vi "AutoROI_Setting_UI.vi"(6 "Root":path, 7 "ProjectName":string, 8 "error in (no error)":errorcluster, 11 "Vision_Image":T4(plugin-control)) -> (0 "error out":errorcluster)   [LabVIEW 2019]
uses:
  Controls/AutoROIUI.ctl
  <vilib>/Utility/miscctls.llb/LVPointTypeDef.ctl
  Controls/AutoROIMode.ctl
  <vilib>/vision/Image Controls.llb/IMAQ Image.ctl
  Controls/ROI_List_Action.ctl
  Controls/AutoROIPage.ctl
panel:
  in  "ReadImage":bool
  in  "ROI List":i32[](listbox)
  out "ModeTab":T1
  in  "Numbers":i32=1 min=1 step=1
  in  "ROIDim":T2={"X Pitch"=200, "X Numbers"=1, "Y Pitch"=150, "Y Numbers"=1} {"X Pitch" min=1 step=1; "X Numbers" min=1 step=1; "Y Numbers" min=1 step=1; "Y Pitch" min=1 step=1}
  in  "Step":i32(ring)=1 items=["1 pixel"=1, "10 pixel"=10, "100 pixel"=100]
  in  "X+":bool
  in  "X-":bool
  in  "Y-":bool
  in  "Y+":bool
  in  "Add":bool
  in  "Mode":T3
  in  "Cancel":bool
  in  "OK":bool
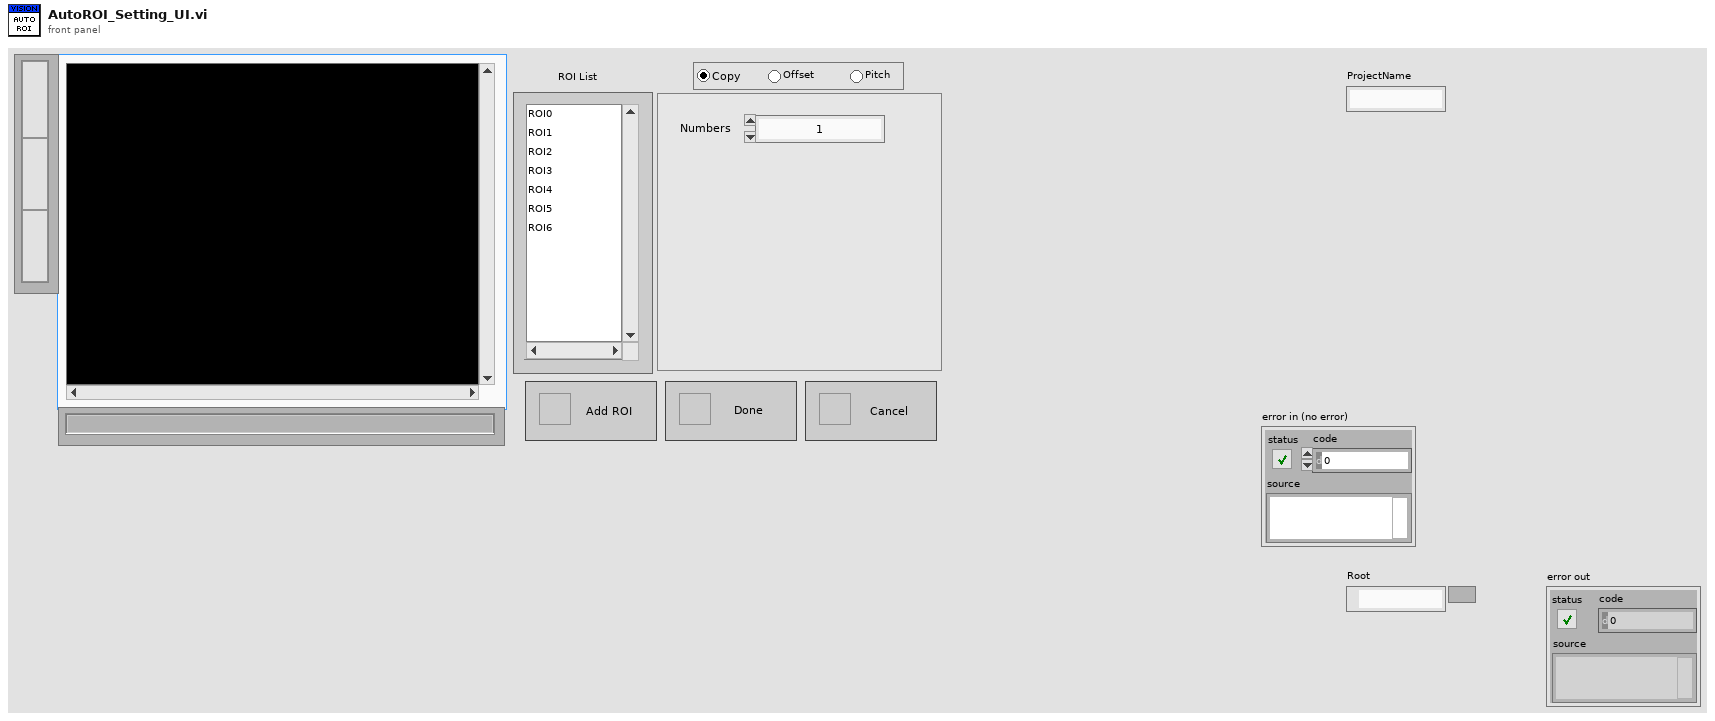
[diagram p1: front panel]
types:
  T1 = typedef "AutoROIPage.ctl" = enum32{"Copy", "Pitch", "Offset"}
  T2 = cluster{"X Pitch":i32, "X Numbers":i32, "Y Pitch":i32, "Y Numbers":i32}
  T3 = typedef "AutoROIMode.ctl" = enum32{"Copy", "Pitch", "Offset"}
  T4 = typedef "IMAQ Image.ctl" = refnum<image>
  T5 = typedef "LVPointTypeDef.ctl" = cluster{"Horizontal":i16, "Vertical":i16}
  T6 = typedef "AutoROIUI.ctl" = cluster{"Message":enum16{"Initialize", "UpdateROIList", "UpdateROI", "Add", "Move", "OK", "Cancel", "Exit"}, "Data":variant}
  T7 = enum8{"Enabled", "Disabled", "Disabled and Grayed Out"}
  T8 = typedef "ROI_List_Action.ctl" = enum16{"Init", "Add ROI", "Delete ROI", "Get All ROI", "Get Specific ROI", "Set Analysis Setting", "Set Process Setting", "Replace All Entries", "ROIEntryBackup", "ROIEntryBackupClear", "ROIEntryReturn"}
  T9 = cluster{"ID":enum32{"External", "Internal"}, "Type":i32, "Coordinates":i32[]}
  T10 = typedef "ROI Descriptor" = cluster{"Global Rectangle":i32[], "Contours":cluster{"ID":enum32{"External", "Internal"}, "Type":u32, "Coordinates":i32[]}[]}
  T11 = enum16{"Initialize", "UpdateROIList", "UpdateROI", "Add", "Move", "OK", "Cancel", "Exit"}
  T12 = typedef "Image Type" = u32
  T13 = typedef "Vision_DataEntry.ctl" = cluster{"vROIName":string, "vROIContour":cluster{"Contour Type":u32, "ROI Type":u32, "Points":i32[]}, "ProcessSetting":T14[], "Analysis_Setting":T16}
  T14 = typedef "Process_Setting.ctl" = cluster{"Enum_PreProcess":T15, "Parameter":string}
  T15 = typedef "VisionProcessName.ctl" = enum16{"*CamParameter*", "CamAttributes", "*Preprocess*", "CG_Brightness", "C_Plane Extraction", "C_Threshold", "G_Lookup Table", "G_Threshold"}
  T16 = typedef "Analysis_Setting.ctl" = cluster{"PreProcess":T17, "Parameter":string}
  T17 = typedef "VisionProcessName.ctl" = enum16{"*CamParameter*", "CamAttributes", "*Preprocess*", "CG_Brightness", "C_Plane Extraction", "C_Threshold", "G_Lookup Table", "G_Threshold", "B_Image Inversion", "*Algorithm*", "CG_Histogram", "C_Color Matching", "C_Color Pattern Matching", "G_PatternMatch", "CG_Find Straight Edge", "CG_Adv. Find Straight Edge", "CG_Find Circular Edge", "G_Max Clamp", "G_Clamp (Rake)", "G_Pattern Matching"}
  T18 = cluster{"Points[0]":i32, "Points[1]":i32, "Points[2]":i32, "Points[3]":i32}
  T19 = cluster{"ID":enum32{"External", "Internal"}, "Type":i32, "Coordinates":i32[]}[]
  T20 = typedef "Vision_DataEntry.ctl" = cluster{"vROIName":string, "vROIContour":cluster{"Contour Type":u32, "ROI Type":u32, "Points":i32[]}, "ProcessSetting":T14[], "Analysis_Setting":T21}
  T21 = typedef "Analysis_Setting.ctl" = cluster{"PreProcess":T22, "Parameter":string}
  T22 = typedef "V_Analysis_Type.ctl" = enum16{"None", "C_Color Pattern Matching", "G_PatternMatching", "G_ShapeDectect", "G_GeometricMatch", "B_Area Check"}
  T23 = cluster{"ID":enum32{"External", "Internal"}, "Type":u32, "Coordinates":i32[]}[]
  T24 = cluster{"ID":enum32{"External", "Internal"}, "Type":u32, "Coordinates":i32[]}
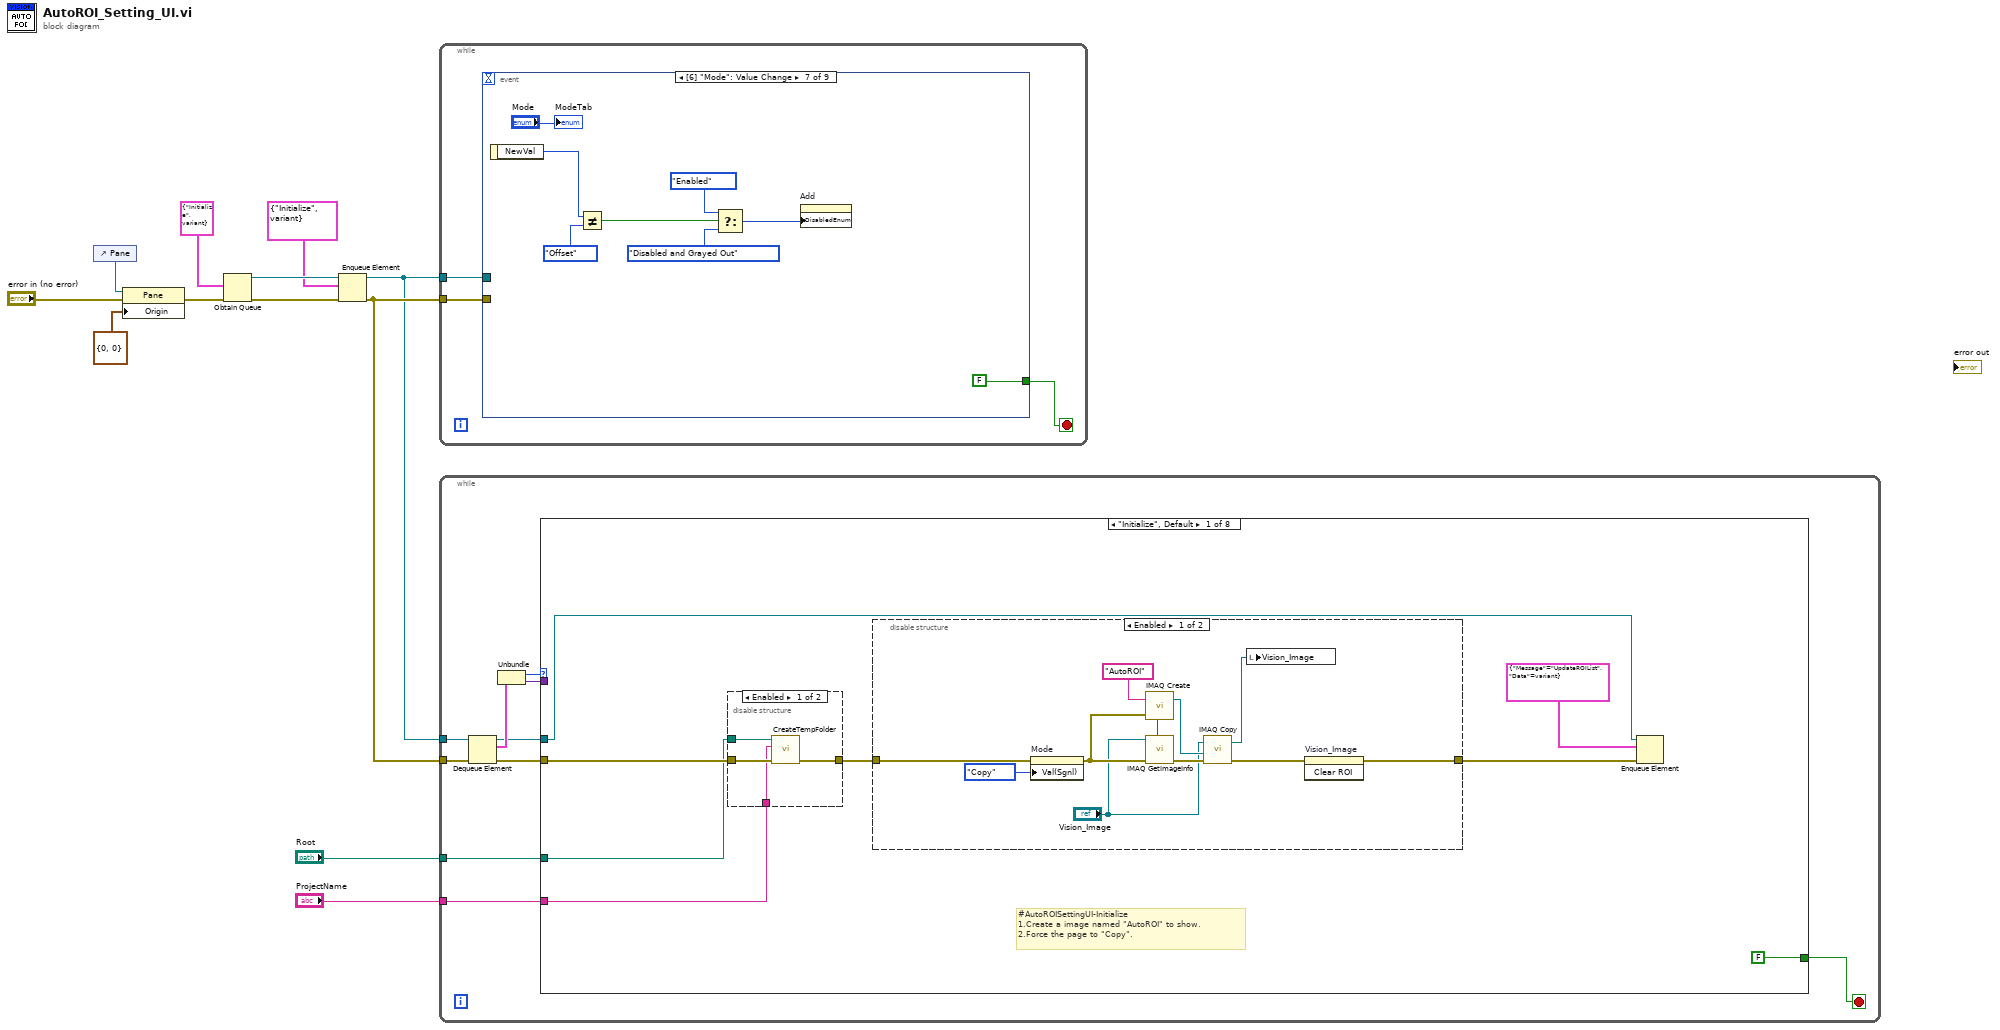
[diagram p0: block diagram]
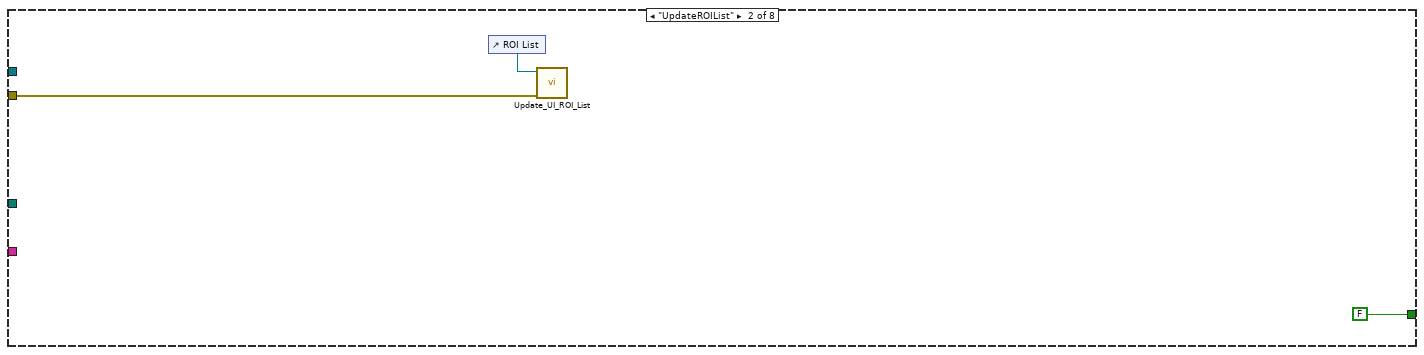
[diagram p4: hidden frame]
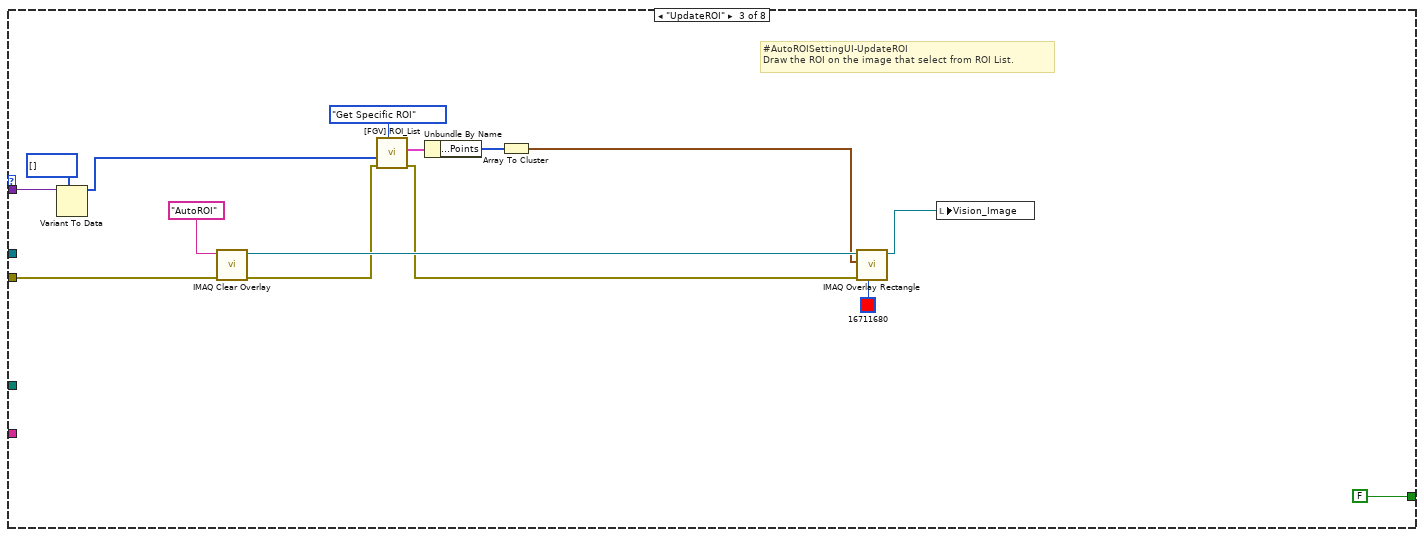
[diagram p5: hidden frame]
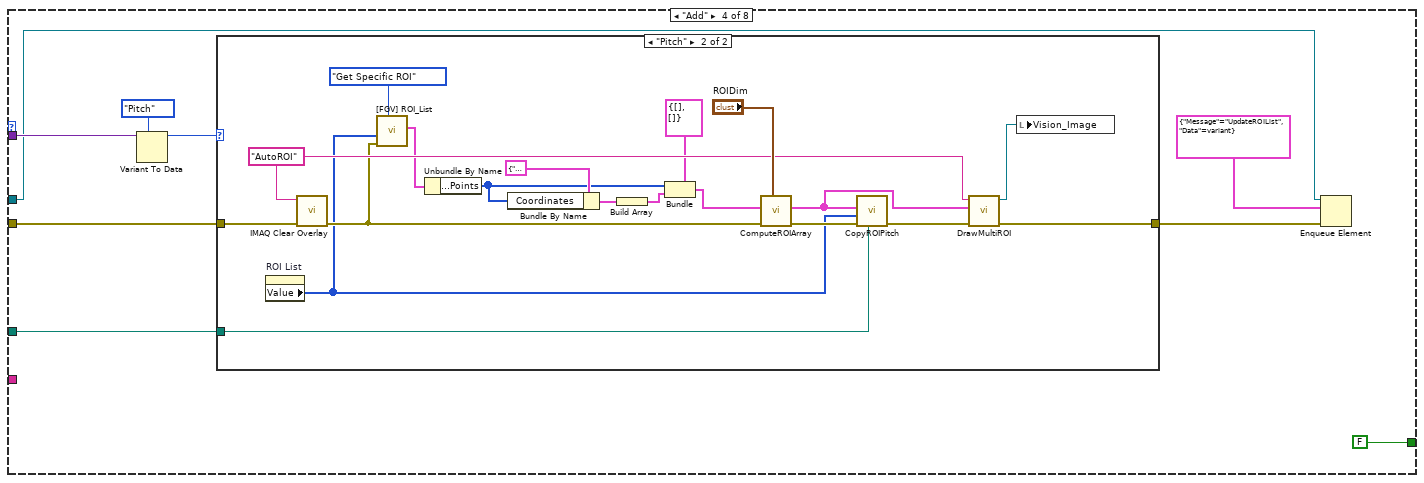
[diagram p6: hidden frame]
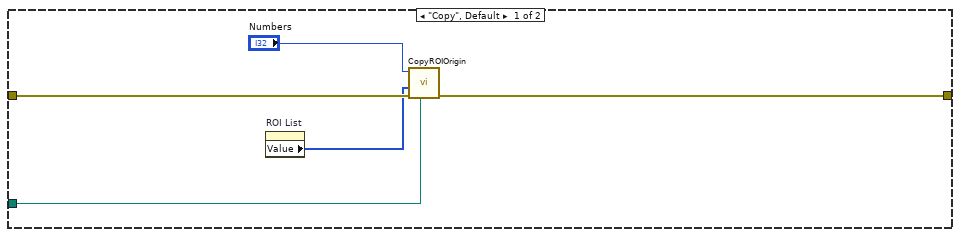
[diagram p7: hidden frame]
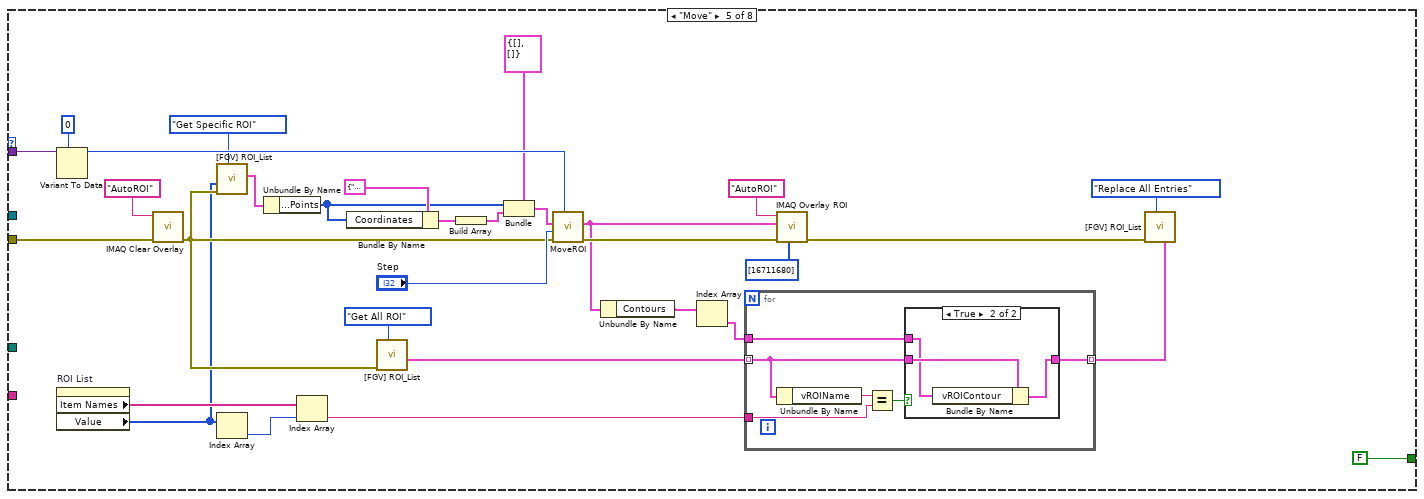
[diagram p8: hidden frame]
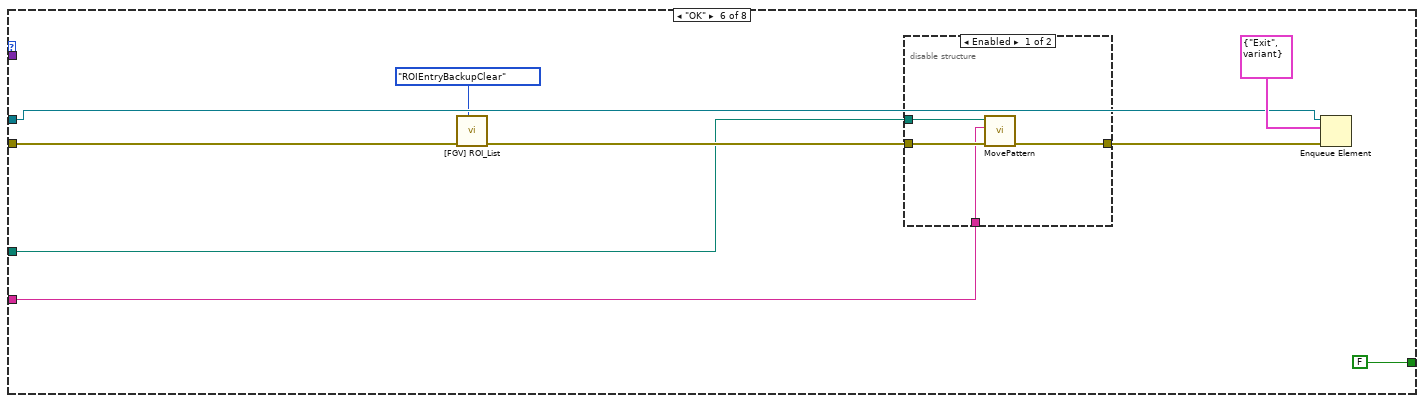
[diagram p10: hidden frame]
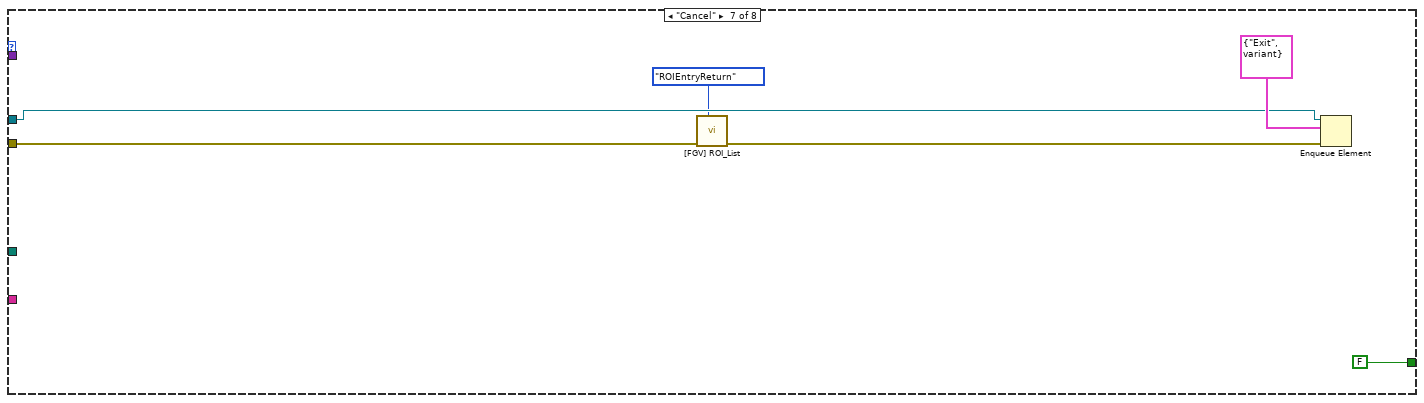
[diagram p12: hidden frame]
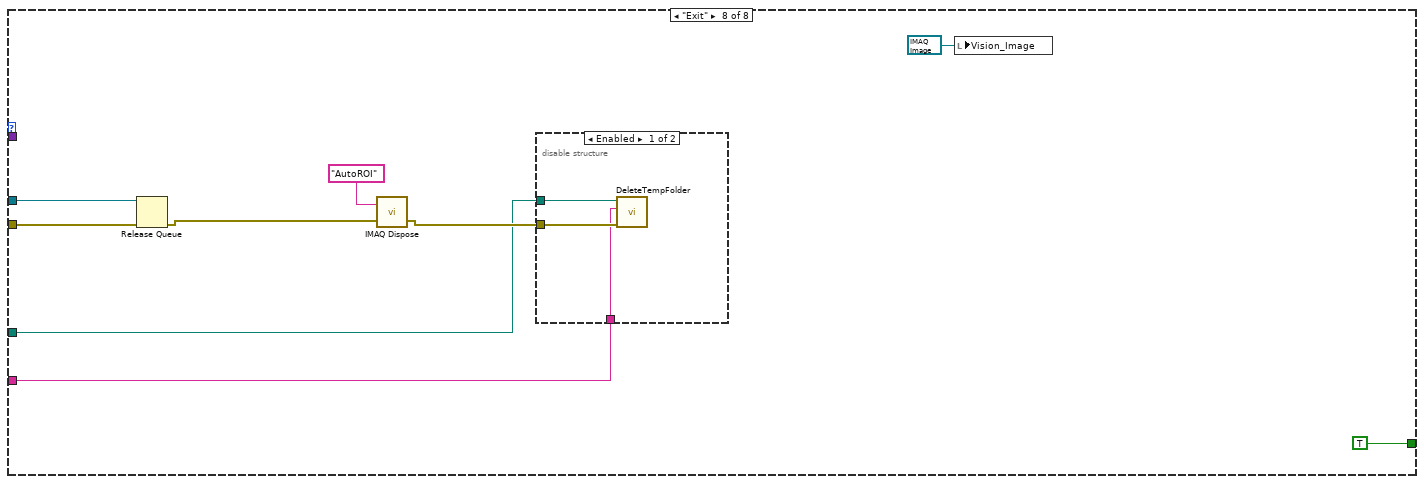
[diagram p13: hidden frame]
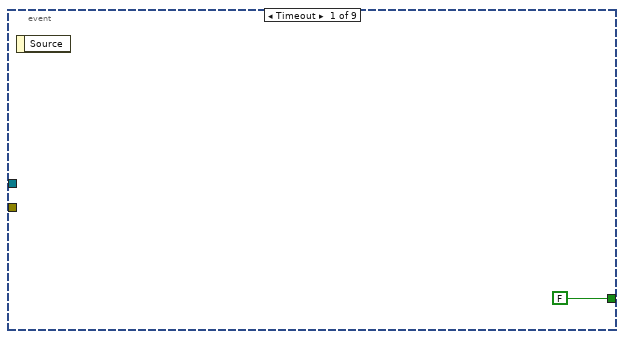
[diagram p15: hidden frame]
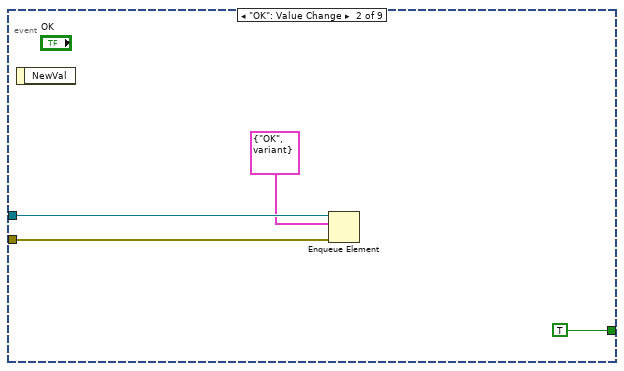
[diagram p16: hidden frame]
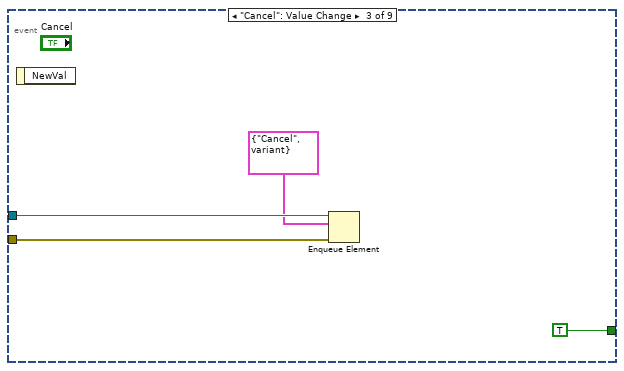
[diagram p17: hidden frame]
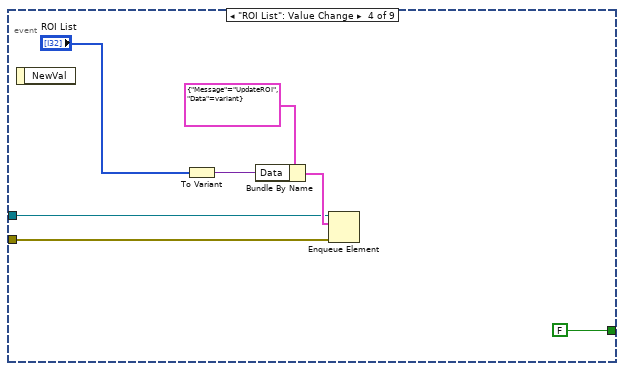
[diagram p18: hidden frame]
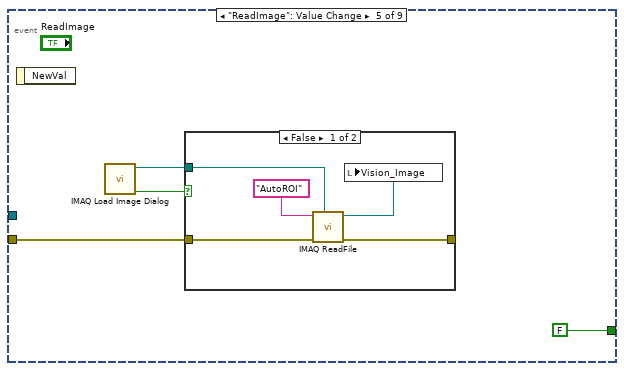
[diagram p19: hidden frame]
diagram:
  n1 = control-ref of="Pane"() -> (w6:refnum<vi>)
  n2 = property class="Pane"(reference=w6, error in="error in (no error)", "Origin"=T5 {"Horizontal"=0, "Vertical"=0}) -> (error out=w5:errorcluster)  [unwired: 1 out]
  n3 = Obtain Queue(element data type=T6 {"Message"=enum."Initialize", "Data"=variant} ("AutoROIUI"), error in (no error)=w5) -> (queue out=w12:refnum<queue>, error out=w11:errorcluster)  [unwired: 3 in, 1 out]
  n4 = Enqueue Element(queue=w12, element=T6 {"Message"=enum."Initialize", "Data"=variant}, error in (no error)=w11) -> (queue out=w7:refnum<queue>, error out=w8:errorcluster)  [unwired: 1 in, 1 out]
  n5 = while {
    tunnel: w7 -> [w14]
    tunnel: w8 -> [w13]
    stop <- w15 stop-if-true
    n6 = event shown="[6] \"Mode\": Value Change" {
      selector: _ -> [_ _ _ _ _ _ _ _ _]
      dyn-events: _ -> [_ _ _ _ _ _ _ _ _]
      timeout: _ -> [_ _ _ _ _ _ _ _ _]
      tunnel: [FALSE TRUE TRUE FALSE FALSE _ FALSE FALSE FALSE] -> w15
      tunnel: w14 -> [_ w19 w23 w27 _ w43 _ w65 w73]
      tunnel: w13 -> [_ w18 w22 w26 w33 w42 _ w64 w72]
      event Timeout {
        n7 = event-data() -> ()  [unwired: 1 in, 1 out]
      }
      event "OK": Value Change {
        n8 = event-data() -> ()  [unwired: 1 in, 1 out]
        n9 = Enqueue Element(queue=w19, element=T6 {"Message"=enum."OK", "Data"=variant}, error in (no error)=w18) -> ()  [unwired: 1 in, 3 out]
      }
      event "Cancel": Value Change {
        n10 = event-data() -> ()  [unwired: 1 in, 1 out]
        n11 = Enqueue Element(queue=w23, element=T6 {"Message"=enum."Cancel", "Data"=variant}, error in (no error)=w22) -> ()  [unwired: 1 in, 3 out]
      }
      event "ROI List": Value Change {
        n12 = event-data() -> ()  [unwired: 1 in, 1 out]
        n13 = To Variant(anything="ROI List") -> (Variant=w29:variant)
        n14 = Bundle By Name(cluster=T6 {"Message"=enum."UpdateROI", "Data"=variant} ("element"), "Data"=w29) -> (w28:T6)
        n15 = Enqueue Element(queue=w27, element=w28, error in (no error)=w26) -> ()  [unwired: 1 in, 3 out]
      }
      event "ReadImage": Value Change {
        n16 = event-data() -> ()  [unwired: 1 in, 1 out]
        n17 = call "IMAQ Load Image Dialog"() -> ("Cancelled?"=w35:bool, "Path"=w34:path)  [unwired: 9 in, 1 out]
        n18 = case shown="False" w35 {
          tunnel: w33 -> [w40 w41]
          tunnel: [w39 w41] -> _
          tunnel: w34 -> [w37 _]
          frame False {
            n19 = call "IMAQ ReadFile"("File Path"=w37, "error in (no error)"=w40, "Image"="AutoROI" ("Image Name")) -> ("error out"=w39:errorcluster, "Image Out"=w36:T4)  [unwired: 4 in, 3 out]
            n20 = local write "Vision_Image"(w36) -> ()
          }
          frame True {
          }
        }
      }
      event "Vision_Image": Mouse Up {
        w45 = i32[] [2] items=["No Event"=0, "Click Event"=1, "Draw Event"=2, "Size Event"=4, "Scroll Event"=5, "Double Click Event"=8] ("Which Events")
        n21 = event-data() -> ()  [unwired: 1 in, 1 out]
        n22 = invoke on="Vision_Image" class="ImageControl" method="Get Last Event"("Which Events"=w45) -> ("Type"=w46:i32)  [unwired: 7 in, 7 out]
        n23 = Not Equal To 0?(x=w46) -> (x != 0?=w44:bool)
        n24 = case shown="True" w44 {
          tunnel: w43 -> [_ w51]
          tunnel: w42 -> [w47 w50]
          tunnel: [w47 w49] -> _
          frame False {
          }
          frame True {
            n25 = Enqueue Element(queue=w51, element=T6 {"Message"=enum."UpdateROI", "Data"=variant}, error in (no error)=w50) -> (error out=w49:errorcluster)  [unwired: 1 in, 2 out]
          }
        }
      }
      event Value Change {
        n26 = event-data() -> ("NewVal"=w55:T3)  [unwired: 1 in]
        n27 = Not Equal?(x=w55, y=AutoROIMode."Offset") -> (x != y?=w56:bool)
        n28 = Select(t=T7."Enabled" ("Disabled"), s=w56, f=T7."Disabled and Grayed Out" ("Disabled")) -> (s? t:f=w52:T7)
        n29 = property on="Add" class="Bool"("DisabledEnum"=w52) -> ()  [unwired: 2 in, 2 out]
        "ModeTab" <- "Mode"
      }
      event "Add": Value Change {
        n30 = event-data() -> ()  [unwired: 1 in, 1 out]
        n31 = local read "Mode"() -> (w63:T3)
        n32 = To Variant(anything=w63) -> (Variant=w61:variant)
        n33 = Bundle By Name(cluster=T6 {"Message"=enum."Add", "Data"=variant} ("element"), "Data"=w61) -> (w60:T6)
        n34 = Enqueue Element(queue=w65, element=w60, error in (no error)=w64) -> ()  [unwired: 1 in, 3 out]
      }
      event "X+", "X-", "Y+", "Y-": Value Change {
        n35 = event-data() -> ()  [unwired: 1 in, 1 out]
        n36 = Build Array("X+", "X-", "Y+", "Y-") -> (w75:bool[])
        n37 = Search 1D Array(1D array=w75, element=TRUE) -> (index of element=w69:i32)  [unwired: 1 in]
        n38 = To Variant(anything=w69) -> (Variant=w68:variant)
        n39 = Bundle By Name(cluster=T6 {"Message"=enum."Move", "Data"=variant} ("element"), "Data"=w68) -> (w70:T6)
        n40 = Enqueue Element(queue=w73, element=w70, error in (no error)=w72) -> ()  [unwired: 1 in, 3 out]
      }
    }
  }
  n41 = while {
    tunnel: w8 -> [w89]
    tunnel: w7 -> [w88]
    tunnel: "Root" -> [w81]
    tunnel: "ProjectName" -> [w80]
    stop <- w82 stop-if-true
    n42 = Dequeue Element(queue=w88, error in (no error)=w89) -> (queue out=w85:refnum<queue>, element=w87:T6, error out=w84:errorcluster)  [unwired: 1 in, 1 out]
    n43 = Unbundle(w87) -> ("Message"=w86:T11, "Data"=w83:variant)
    n44 = case shown="\"Initialize\", Default" w86 {
      tunnel: [FALSE FALSE FALSE FALSE FALSE FALSE FALSE TRUE] -> w82
      tunnel: w85 -> [w91 _ _ w132 _ w212 w222 w232]
      tunnel: w84 -> [w96 w114 w121 w139 w193 w211 w221 w231]
      tunnel: w83 -> [_ _ w123 w138 w194 _ _ _]
      tunnel: w81 -> [w90 _ _ w135 _ w206 _ w225]
      tunnel: w80 -> [w94 _ _ _ _ w207 _ w226]
      frame "Initialize", Default {
        # "#AutoROISettingUI-Initialize\n1.Create a image named \"AutoROI\" to show.\n2.Force the page to \"Copy\"."
        n45 = disable-structure shown="Enabled" {
          disable-tunnel: w96 -> [w101 w102]
          disable-tunnel: [w100 w102] -> w95
          disable-tunnel: w94 -> [w99 _]
          disable-tunnel: w90 -> [w98 _]
          frame Enabled {
            n46 = call "CreateTempFolder.vi"("error in (no error)"=w101, "Project"=w99, "Root In"=w98) -> ("error out"=w100:errorcluster)  [unwired: 7 in, 1 out]
          }
          frame Disabled {
          }
        }
        n47 = disable-structure shown="Enabled" {
          disable-tunnel: w95 -> [w113 _]
          disable-tunnel: [w103 _] -> w92
          frame Enabled {
            n48 = property on="Mode" class="RadioBtnsControl (strict)"(error in=w113, "Val(Sgnl)"=AutoROIMode."Copy" ("Mode")) -> (error out=w109:errorcluster)  [unwired: 1 in, 1 out]
            n49 = call "IMAQ GetImageInfo"("error in (no error)"=w109, "Image"="Vision_Image") -> ("error out"=w107:errorcluster, "Image Type"=w110:T12)  [unwired: 2 in, 6 out]
            n50 = call "IMAQ Create"("Image Name"="AutoROI", "Image Type"=w110, "error in (no error)"=w109) -> ("New Image"=w108:T4)  [unwired: 2 in, 1 out]
            n51 = call "IMAQ Copy"("error in (no error)"=w107, "Image Dst"=w108, "Image Src"="Vision_Image") -> ("error out"=w104:errorcluster, "Image Dst Out"=w105:T4)  [unwired: 3 in]
            n52 = local write "Vision_Image"(w105) -> ()
            n53 = invoke on="Vision_Image" class="ImageControl" method="Clear ROI"(error in=w104) -> (error out=w103:errorcluster)  [unwired: 2 in, 2 out]
          }
          frame Disabled {
          }
        }
        n54 = Enqueue Element(queue=w91, element=T6 {"Message"=enum."UpdateROIList", "Data"=variant}, error in (no error)=w92) -> ()  [unwired: 1 in, 3 out]
      }
      frame "UpdateROIList" {
        n55 = control-ref of="ROI List"() -> (w115:refnum<vi>)
        n56 = call "Update_UI_ROI_List.vi"("error in (no error)"=w114, "LstBox Refnum"=w115) -> ()  [unwired: 9 in, 1 out]
      }
      frame "UpdateROI" {
        # "#AutoROISettingUI-UpdateROI\nDraw the ROI on the image that select from ROI List."
        n57 = Variant To Data(type=i32[] [] ("ROI List 2"), Variant=w123) -> (data=w120:i32[])  [unwired: 1 in, 1 out]
        n58 = call "IMAQ Clear Overlay"("error in (no error)"=w121, "Image"="AutoROI" ("Image Name")) -> ("error out"=w118:errorcluster, "Image Out"=w129:T4)  [unwired: 8 in]
        n59 = call "[FGV] ROI_List.vi"("Action"=ROI_List_Action."Get Specific ROI", "error in (no error)"=w118, "ROIs_Index"=w120) -> ("error out"=w117:errorcluster, "ROI Entry"=w125:T13)  [unwired: 6 in, 1 out]
        n60 = Unbundle By Name(w125) -> ("vROIContour.Points"=w126:i32[])
        n61 = Array To Cluster(array=w126) -> (cluster=w119:T18)
        n62 = call "IMAQ Overlay Rectangle"("Color"=u32 16711680, "error in (no error)"=w117, "Rectangle"=w119, "Image"=w129) -> ("Image Out"=w128:T4)  [unwired: 6 in, 1 out]
        n63 = local write "Vision_Image"(w128) -> ()
      }
      frame "Add" {
        n64 = Variant To Data(type=AutoROIMode."Pitch" ("Mode"), Variant=w138) -> (data=w136:T3)  [unwired: 1 in, 1 out]
        n65 = case shown="\"Pitch\"" w136 {
          tunnel: w139 -> [w145 w163]
          tunnel: w135 -> [w143 w157]
          tunnel: [w141 w146] -> w133
          frame "Copy", Default {
            n66 = property on="ROI List" class="LstBox (strict)"() -> ("Value"=w142:i32[])  [unwired: 2 in, 2 out]
            n67 = call "CopyROIOrigin.vi"("Root"=w143, "error in (no error)"=w145, "ROI List"=w142, "Numbers"="Numbers") -> ("error out"=w141:errorcluster)  [unwired: 7 in]
          }
          frame "Pitch" {
            w162 = "AutoROI" ("Image Name")
            n68 = property on="ROI List" class="LstBox (strict)"() -> ("Value"=w148:i32[])  [unwired: 2 in, 2 out]
            n69 = call "IMAQ Clear Overlay"("error in (no error)"=w163, "Image"=w162) -> ("error out"=w149:errorcluster)  [unwired: 8 in, 1 out]
            n70 = call "[FGV] ROI_List.vi"("Action"=ROI_List_Action."Get Specific ROI", "error in (no error)"=w149, "ROIs_Index"=w148) -> ("ROI Entry"=w155:T13)  [unwired: 6 in, 2 out]
            n71 = Unbundle By Name(w155) -> ("vROIContour.Points"=w152:i32[])
            n72 = Bundle By Name(cluster=T9 {"ID"=enum."External", "Type"=3, "Coordinates"=[]}, "Coordinates"=w152) -> (w151:T9)
            n73 = Build Array(w151) -> (w150:T19)
            n74 = Bundle(cluster=T10 {"Global Rectangle"=[], "Contours"=[]} ("ROI Descriptor"), "Global Rectangle"=w152, "Contours"=w150) -> (w147:T10)
            n75 = call "ComputeROIArray.vi"("ROIDim"="ROIDim", "error in (no error)"=w149, "ROI In"=w147) -> ("error out"=w158:errorcluster, "ROIs Out"=w160:T10[])  [unwired: 7 in]
            n76 = call "CopyROIPitch.vi"("Root"=w157, "error in (no error)"=w158, "ROI List"=w148, "ROIs"=w160) -> ("error out"=w159:errorcluster)  [unwired: 7 in]
            n77 = call "DrawMultiROI.vi"("error in (no error)"=w159, "ROIs"=w160, "Image In"=w162) -> ("error out"=w146:errorcluster, "Image Out"=w161:T4)  [unwired: 7 in]
            n78 = local write "Vision_Image"(w161) -> ()
          }
        }
        n79 = Enqueue Element(queue=w132, element=T6 {"Message"=enum."UpdateROIList", "Data"=variant}, error in (no error)=w133) -> ()  [unwired: 1 in, 3 out]
      }
      frame "Move" {
        n80 = Variant To Data(type=0 ("index of element"), Variant=w194) -> (data=w191:i32)  [unwired: 1 in, 1 out]
        n81 = property on="ROI List" class="LstBox (strict)"() -> ("Item Names"=w173:string[], "Value"=w165:i32[])  [unwired: 2 in, 2 out]
        n82 = call "IMAQ Clear Overlay"("error in (no error)"=w193, "Image"="AutoROI" ("Image Name")) -> ("error out"=w175:errorcluster)  [unwired: 8 in, 1 out]
        n83 = call "[FGV] ROI_List.vi"("Action"=ROI_List_Action."Get Specific ROI", "error in (no error)"=w175, "ROIs_Index"=w165) -> ("ROI Entry"=w182:T13)  [unwired: 6 in, 2 out]
        n84 = Index Array(array=w165) -> (element=w172:i32)  [unwired: 1 in]
        n85 = Unbundle By Name(w182) -> ("vROIContour.Points"=w179:i32[])
        n86 = Index Array(array=w173, index=w172) -> (element=w171:string)
        n87 = Bundle By Name(cluster=T9 {"ID"=enum."External", "Type"=3, "Coordinates"=[]}, "Coordinates"=w179) -> (w177:T9)
        n88 = call "[FGV] ROI_List.vi"("Action"=ROI_List_Action."Get All ROI", "error in (no error)"=w175) -> ("All ROI"=w174:T20[])  [unwired: 7 in, 2 out]
        n89 = Build Array(w177) -> (w176:T19)
        n90 = Bundle(cluster=T10 {"Global Rectangle"=[], "Contours"=[]} ("ROI Descriptor"), "Global Rectangle"=w179, "Contours"=w176) -> (w178:T10)
        n91 = call "MoveROI.vi"("Direction"=w191, "error in (no error)"=w175, "Pitch"="Step", "ROI In"=w178) -> ("error out"=w190:errorcluster, "ROI Out"=w170:T10)  [unwired: 6 in]
        n92 = Unbundle By Name(w170) -> ("Contours"=w169:T23)
        n93 = Index Array(array=w169) -> (element=w166:T24)  [unwired: 1 in]
        n94 = for {
          tunnel: w174 -> [w196] mode=indexing
          tunnel: w171 -> [w200]
          tunnel: w166 -> [w197]
          tunnel: [w198] -> w167 mode=indexing
          n95 = Unbundle By Name(w196) -> ("vROIName"=w201:string)
          n96 = Equal?(x=w201, y=w200) -> (x = y?=w199:bool)
          n97 = case shown="True" w199 {
            tunnel: [w202 w203] -> w198
            tunnel: w196 -> [w202 w205]
            tunnel: w197 -> [_ w204]
            frame False {
            }
            frame True {
              n98 = Bundle By Name(cluster=w205, "vROIContour"=w204) -> (w203:T20)
            }
          }
        }
        n99 = call "IMAQ Overlay ROI"("Colors (Green)"=u32[] [16711680], "error in (no error)"=w190, "ROI Descriptor"=w170, "Image"="AutoROI" ("Image Name")) -> ("error out"=w168:errorcluster)  [unwired: 6 in, 1 out]
        n100 = call "[FGV] ROI_List.vi"("ROIEntriesIn"=w167, "Action"=ROI_List_Action."Replace All Entries", "error in (no error)"=w168) -> ()  [unwired: 6 in, 3 out]
      }
      frame "OK" {
        n101 = call "[FGV] ROI_List.vi"("Action"=ROI_List_Action."ROIEntryBackupClear", "error in (no error)"=w211) -> ("error out"=w209:errorcluster)  [unwired: 7 in, 2 out]
        n102 = disable-structure shown="Enabled" {
          disable-tunnel: w209 -> [w218 w219]
          disable-tunnel: [w217 w219] -> w208
          disable-tunnel: w207 -> [w216 _]
          disable-tunnel: w206 -> [w215 _]
          frame Enabled {
            n103 = call "MovePattern.vi"("error in (no error)"=w218, "Project"=w216, "Root In"=w215) -> ("error out"=w217:errorcluster)  [unwired: 7 in, 1 out]
          }
          frame Disabled {
          }
        }
        n104 = Enqueue Element(queue=w212, element=T6 {"Message"=enum."Exit", "Data"=variant}, error in (no error)=w208) -> ()  [unwired: 1 in, 3 out]
      }
      frame "Cancel" {
        n105 = call "[FGV] ROI_List.vi"("Action"=ROI_List_Action."ROIEntryReturn") -> ()  [unwired: 8 in, 3 out]
        n106 = Enqueue Element(queue=w222, element=T6 {"Message"=enum."Exit", "Data"=variant}, error in (no error)=w221) -> ()  [unwired: 1 in, 3 out]
      }
      frame "Exit" {
        n107 = Release Queue(queue=w232, error in (no error)=w231) -> (error out=w229:errorcluster)  [unwired: 1 in, 2 out]
        n108 = call "IMAQ Dispose"("Image"="AutoROI" ("Image Name"), "error in (no error)"=w229) -> ("error out"=w227:errorcluster)  [unwired: 4 in]
        n109 = disable-structure shown="Enabled" {
          disable-tunnel: w227 -> [w236 _]
          disable-tunnel: w226 -> [w235 _]
          disable-tunnel: w225 -> [w234 _]
          frame Enabled {
            n110 = call "DeleteTempFolder.vi"("error in (no error)"=w236, "Project"=w235, "Root"=w234) -> ()  [unwired: 8 in, 1 out]
          }
          frame Disabled {
          }
        }
        n111 = local write "Vision_Image"(T4 refnum ("Vision_Image")) -> ()
      }
    }
  }
